vi "Update Build Spec Version.vi"(8 "error in (no error)":errorcluster, 9 "Version":T1, 10 "Search Pattern":string, 11 "LabVIEW Build Script in":refnum<class "LabVIEW Build Script.lvclass">) -> (0 "error out":errorcluster)   [LabVIEW 2021, in "LabVIEW Build Script.lvclass"]
uses:
  LabVIEW Build Script.lvclass
  <vilib>/CIF Foundation/CIF LabVIEW Scripting/LV Scripting/Typedef/Version.ctl
  LabVIEW Build Script.lvclass/LabVIEW Build Script.ctl
  Build Script Common/Typedef/Build Script Errors.ctl
  <vilib>/CIF Foundation/CIF Utilities/Errors/Append Error Location.vi
  Build Script Common/Build Script Common.lvlib
  <vilib>/CIF Foundation/CIF LabVIEW Scripting/LV Scripting/LV Scripting Utilities.lvlib
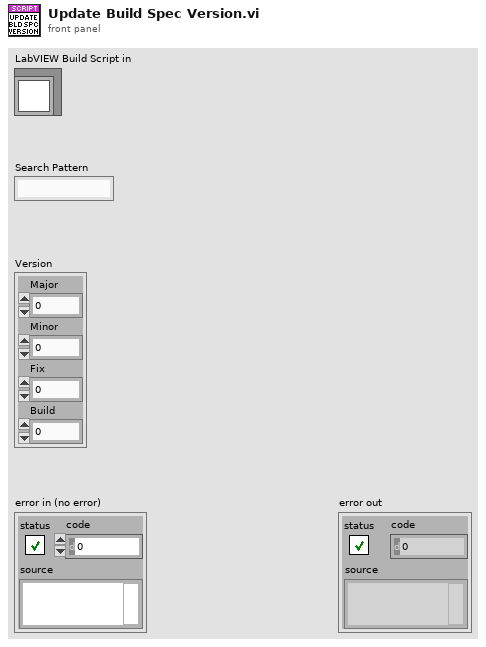
[diagram p1: front panel]
types:
  T1 = typedef "Version.ctl" = cluster{"Major":u16, "Minor":u16, "Fix":u16, "Build":u16}
  T2 = typedef "Build Script Common.lvlib/Build Script Errors.ctl" = enum16{"Item not found"}
  T3 = typedef "LV Scripting Utilities.lvlib/BuildSpec Map.ctl" = map{string, refnum<vi>}
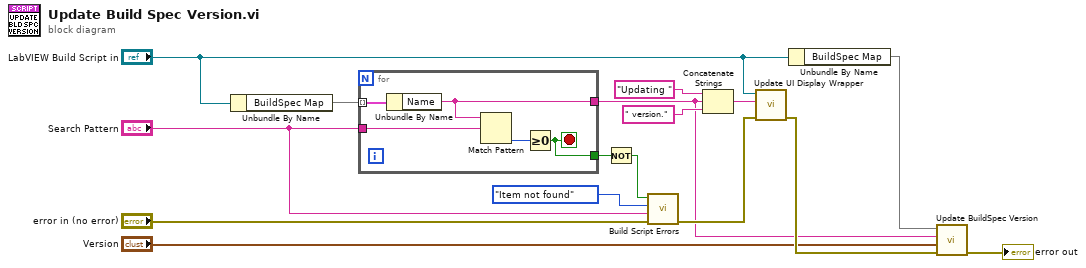
[diagram p0: block diagram]
diagram:
  n1 = Unbundle By Name("LabVIEW Build Script in") -> ("BuildSpec Map"=w13:T3)
  n2 = for {
    tunnel: w13 -> [w21] mode=indexing
    tunnel: "Search Pattern" -> [w20]
    tunnel: [w18] -> w1
    tunnel: [w17] -> w11
    stop <- w17 stop-if-true
    n3 = Unbundle By Name(w21) -> ("Name"=w18:string)
    n4 = Match Pattern(string=w18, regular expression=w20) -> (offset past match=w19:i32)  [unwired: 1 in, 3 out]
    n5 = Greater Or Equal To 0?(x=w19) -> (x >= 0?=w17:bool)
  }
  n6 = Not(x=w11) -> (.not. x?=w10:bool)
  n7 = call "Build Script Errors.vi"("error in (no error)"="error in (no error)", "String to Append"="Search Pattern", "Error"=Build_Script_Errors."Item not found", "Insert Error"=w10) -> ("error out"=w6:errorcluster)  [unwired: 7 in]
  n8 = Concatenate Strings("Updating " ("Update for Display"), w1, " version." ("string")) -> (w15:string)
  n9 = call "Update UI Display Wrapper.vi"("error in (no error)"=w6, "Update for Display"=w15, "LabVIEW Build Script in"="LabVIEW Build Script in") -> ("error out"=w4:errorcluster)  [unwired: 8 in]
  n10 = Unbundle By Name("LabVIEW Build Script in") -> ("BuildSpec Map"=w5:T3)
  n11 = call <vilib>:"Update BuildSpec Version.vi"("error in (no error)"=w4, "New Version"="Version", "BuildSpec Name"=w1, "BuildSpec Map"=w5) -> ("error out"=→"error out":errorcluster)  [unwired: 7 in]
